vi "GetProbePlanCoordinates.vi"(1 "Probe Card Channels":i32=32) -> (0 "file path":string, 2 "OK?":bool, 3 "Array":T1(array[cluster]))   [LabVIEW 2018]
doc: "Utility to read probe plan from text file and generate respective coordinates in global variable."
uses:
  general_VIs/globals/QC_MeasurementSetup.vi
  ProbePlanParams.vi
  <vilib>/regexp/Match Regular Expression.xnode
panel:
  out "No. probe points":string
  in  "ProbePoints":T2
  out "String":string
  in  "Stop Button":bool
  in  "OK Button":bool
  in  "Region":u16(ring)
  out "Coordinates":string[][](table)
  # "ProbePlan Coordinates"
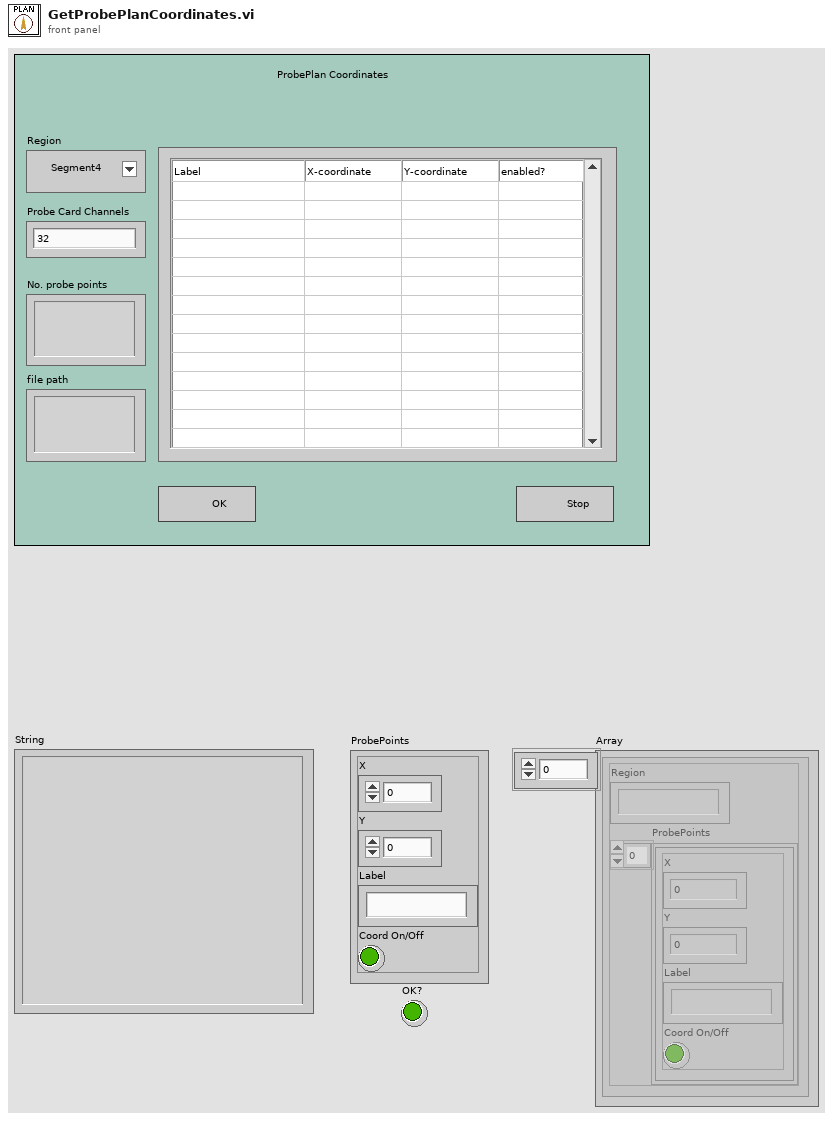
[diagram p1: front panel]
types:
  T1 = cluster{"Region":string, "ProbePoints":cluster{"X":dbl, "Y":dbl, "Label":string, "Coord On/Off":bool}[]}[]
  T2 = cluster{"X":dbl, "Y":dbl, "Label":string, "Coord On/Off":bool}
  T3 = cluster{"Region":string, "ProbePoints":cluster{"X":dbl, "Y":dbl, "Label":string, bool}[]}[]
  T4 = enum16{"open", "replace", "create", "open or create", "replace or create", "replace or create with confirmation"}
  T5 = cluster{"X":dbl, "Y":dbl, "Label":string, bool}[]
  T6 = cluster{"Bias Supply":refnum<class "SupplyControl.lvclass">, "SMU":refnum<class "SupplyControl.lvclass">, "LCR":refnum<class "LCRControl.lvclass">, "ProbeStation":refnum<class "ProbeStationControl.lvclass">, "Arduino":refnum<class "ArduinoControl.lvclass">, "Measurement switch":refnum<class "Switching.lvclass">, "Probe Card Channels":i32, "Bias Voltage [V]":dbl, "First strip":i32, "Last strip":i32, "Base Voltage [V]":dbl, "Base Ramp Step [V]":dbl, "Base Ramp Interval [ms]":u32, "High Voltage [V]":dbl, "High Ramp Step [V]":dbl, "High Ramp Interval [ms]":u32, "AC frequency [Hz]":i32, "AC amplitude [V]":dbl, "RC Configuration":u16, "Single Needle":bool, "Temperature Readout":enum16{"Read Arduino", "Enter manually"}, "Fraction of good strips [%]":dbl, "Measurement switch used?":bool, "Matrix X Channels":cluster{"Mux1 C1":i32, "Mux1 C2":i32, "Mux2 C1":i32, "Mux2 C2":i32}, "Pinholes Y/N":bool, "Capacitance Y/N":bool, "Resistance Y/N":bool, "Bias Supply Name":string, "SMU Name":string, "LCR Name":string}
  T7 = cluster{"result string":string, "ProbePoints":cluster{"X":dbl, "Y":dbl, "Label":string, bool}[]}
  T8 = cluster{"result string":string, "ProbePoints":cluster{"X":dbl, "Y":dbl, "Label":string, bool}[]}[]
  T9 = cluster{"Region":string, "ProbePoints":cluster{"X":dbl, "Y":dbl, "Label":string, bool}[]}
  T10 = cluster{"X":dbl, "Y":dbl, "Label":string, "Coord On/Off":bool}[]
  T11 = cluster{"Region":string, cluster{"X":dbl, "Y":dbl, "Label":string, "Coord On/Off":bool}[]}
  T12 = cluster{"Strip Number OUT":i32, "X0":i32, "Y0":i32, "X1":i32, "Y1":i32, "Xref":dbl, "Yref":dbl, "ProbePlan type":u32, "Inner pads offset":ext, "Outer pads offset":ext, "l_inner":ext, "l_outer":ext, "strip numbering":u16, "Device Orientation":ext, "Stagger offset":i32, "Yoffset":dbl, "Strip pitch":dbl, "Fiducail separation":dbl, "Radius":ext, "Relative strip angles":dbl, "Probeplan description":string, "ProbePlan array":cluster{"Region":string, "ProbePoints":cluster{"X":dbl, "Y":dbl, "Label":string, "CardViable?":bool}[]}[], "Test ProbePoints":cluster{"Regions Enabled":bool[], "From index":u32[], "To index":u32[], "Strip length [cm]":dbl[]}}
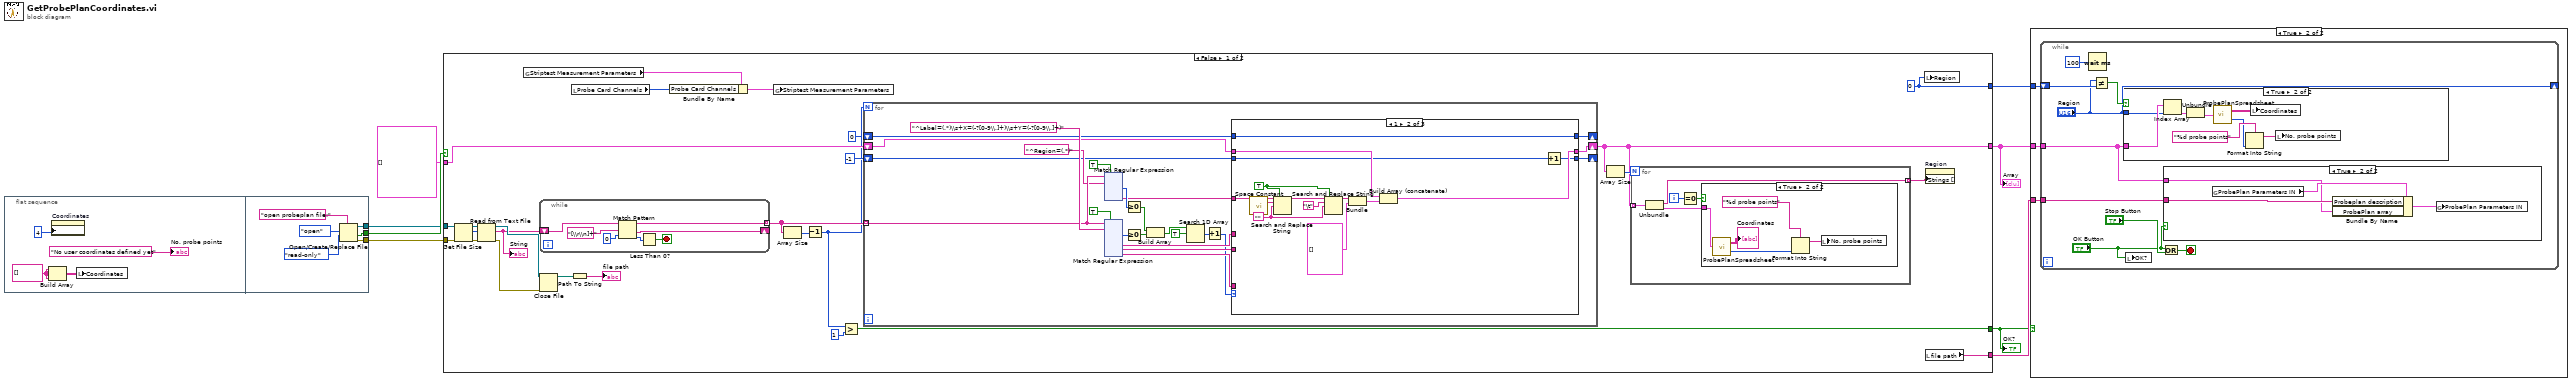
[diagram p0: block diagram]
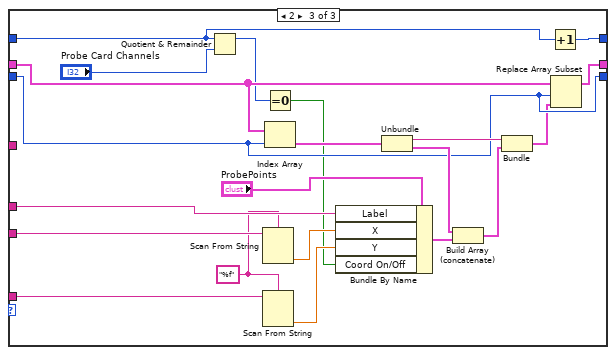
[diagram p7: hidden frame]
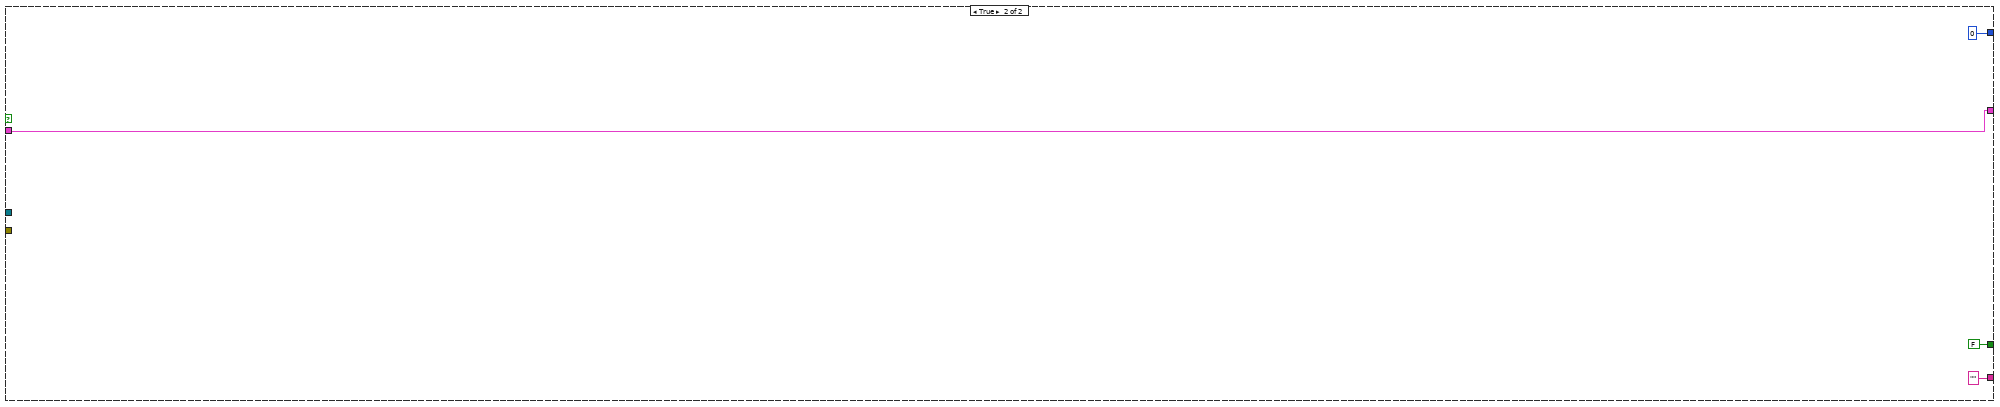
[diagram p8: hidden frame]
diagram:
  n1 = flat-sequence {
    tunnel: [w15] -> w8
    tunnel: [w14] -> w6
    tunnel: [w13] -> w7
    frame #0 {
      w12 = string[] []
      n2 = Build Array(w12, w12, w12) -> (w11:string[][])
      n3 = property on="Coordinates" class="Tbl (strict)"("Number of Columns"=4) -> ()  [unwired: 2 in, 2 out]
      n4 = local write "Coordinates"(w11) -> ()
      "No. probe points" <- "No user coordinates defined yet" ("String 2")
    }
    frame #1 {
      n5 = Open/Create/Replace File(prompt="open probeplan file:", operation (0:open)=T4."open", access (0:read/write)=enum16{"read/write", "read-only", "write-only"}."read-only") -> (refnum out=w13:refnum<file>, cancelled=w15:bool, error out=w14:errorcluster)  [unwired: 3 in]
    }
  }
  n6 = case shown="False" w8 {
    tunnel: T3 [] ("Array") -> [w31 w360]
    tunnel: w7 -> [w44 _]
    tunnel: w6 -> [w39 _]
    tunnel: [w29 w360] -> w4
    tunnel: [w28 0] -> w3
    tunnel: [w24 FALSE] -> w2
    tunnel: [w23 ""] -> w5
    frame False {
      w28 = 0
      n7 = Get File Size(file=w44, error in=w39) -> (refnum out=w43:refnum<file>, size (in bytes)=w38:i64, 0:w41:errorcluster)
      n8 = Read from Text File(file (use dialog)=w43, count=w38, error in=w41) -> (refnum out=w42:refnum<file>, text=w35:string, error out=w40:errorcluster)  [unwired: 1 in, 1 out]
      "String" <- w35
      n9 = global read "QC_MeasurementSetup.vi" "Striptest Measurement Parameters"() -> (w20:T6)
      n10 = while {
        shift-right: [w353] -> _
        shift-left: w35 -> [w356]
        tunnel: [w350] -> w33 mode=indexing
        stop <- w352 stop-if-true
        n11 = Match Pattern(string=w356, regular expression="[\\r\\n]+", offset (0)=0) -> (before substring=w350:string, after substring=w353:string, offset past match=w351:i32)  [unwired: 1 out]
        n12 = Less Than 0?(x=w351) -> (x < 0?=w352:bool)
      }
      n13 = Close File(refnum=w42, error in=w40) -> (path=w37:path)  [unwired: 1 out]
      n14 = Path To String(path=w37) -> (string=→"file path":string)
      n15 = local read "Probe Card Channels"() -> (w21:i32)
      n16 = Bundle By Name(cluster=w20, "Probe Card Channels"=w21) -> (w19:T6)
      n17 = global write "QC_MeasurementSetup.vi" "Striptest Measurement Parameters"(w19) -> ()
      n18 = Array Size(array=w33) -> (size(s)=w34:i32)
      n19 = Decrement(x=w34) -> (x-1=w25:i32)
      n20 = Greater?(x=w25, y=1) -> (0:w24:bool)
      n21 = for {
        N: w25 -> [_]
        tunnel: w33 -> [w71] mode=indexing
        shift-right: [w57] -> _
        shift-left: -1 -> [w58]
        shift-right: [w59] -> w29
        shift-left: w31 -> [w60]
        shift-right: [w56] -> _
        shift-left: 0 -> [w55]
        n22 = xnode "Match Regular Expression"("input string"=w71, "regular expression"="^Region=(.*)", "ignore case? (F)"=TRUE) -> ("offset past match"=w68:i32, "submatch 1"=w61:string)  [unwired: 3 in, 4 out]
        n23 = xnode "Match Regular Expression"("input string"=w71, "regular expression"="^Label=(.*)\\s+X=(-?[0-9\\.]+)\\s+Y=(-?[0-9\\.]+)", "ignore case? (F)"=TRUE) -> ("offset past match"=w74:i32, "submatch 1"=w75:string, "submatch 2"=w72:string, "submatch 3"=w73:string)  [unwired: 3 in, 4 out]
        n24 = Greater Or Equal To 0?(x=w68) -> (x >= 0?=w67:bool)
        n25 = Greater Or Equal To 0?(x=w74) -> (x >= 0?=w66:bool)
        n26 = Build Array(w67, w66) -> (w65:bool[])
        n27 = Search 1D Array(1D array=w65, element=TRUE) -> (index of element=w63:i32)  [unwired: 1 in]
        n28 = Increment(x=w63) -> (x+1=w62:i32)
        n29 = case shown="1" w62 {
          tunnel: w75 -> [_ _ w228]
          tunnel: w73 -> [_ _ w225]
          tunnel: w72 -> [_ _ w227]
          tunnel: w61 -> [_ w203 _]
          tunnel: w60 -> [w196 w209 w220]
          tunnel: [w196 w207 w218] -> w59
          tunnel: w58 -> [w195 w206 w221]
          tunnel: [w195 w205 w221] -> w57
          tunnel: [w194 w204 w212] -> w56
          tunnel: w55 -> [w194 w204 w211]
          frame 0, Default {
          }
          frame 1 {
            w197 = TRUE
            w198 = ""
            n30 = call <vilib>:"Space Constant.vi"() -> ("String"=w202:string)
            n31 = Search and Replace String(replace all?=w197, input string=w203, search string=w202, replace string=w198) -> (result string=w201:string)  [unwired: 4 in, 3 out]
            n32 = Search and Replace String(replace all?=w197, input string=w201, search string="\t", replace string=w198) -> (result string=w200:string)  [unwired: 4 in, 3 out]
            n33 = Bundle("result string"=w200, "ProbePoints"=T5 []) -> (w208:T7)  [unwired: 1 in]
            n34 = Build Array (concatenate)(w209, w208) -> (w207:T8)
            n35 = Increment(x=w206) -> (x+1=w205:i32)
          }
          frame 2 {
            w224 = "%f" ("format string")
            n36 = Quotient & Remainder(x=w211, y="Probe Card Channels") -> (x-y*floor(x/y)=w215:i32)  [unwired: 1 out]
            n37 = Scan From String(format string=w224, input string=w227) -> (output 1=w226:dbl)  [unwired: 3 in, 3 out]
            n38 = Scan From String(format string=w224, input string=w225) -> (output 1=w223:dbl)  [unwired: 3 in, 3 out]
            n39 = Equal To 0?(x=w215) -> (x = 0?=w213:bool)
            n40 = Index Array(array=w220, index=w221) -> (element=w231:T9)
            n41 = Bundle By Name(cluster="ProbePoints", "Label"=w228, "X"=w226, "Y"=w223, "Coord On/Off"=w213) -> (w216:T2)
            n42 = Unbundle(w231) -> ("Region"=w230:string, "ProbePoints"=w229:T5)
            n43 = Build Array (concatenate)(w229, w216) -> (w222:T10)
            n44 = Bundle("Region"=w230, w222) -> (w219:T11)  [unwired: 1 in]
            n45 = Increment(x=w211) -> (x+1=w212:i32)
            n46 = Replace Array Subset(array=w220, new element=w219, index=w221) -> (w218:T3)
          }
        }
      }
      n47 = Array Size(array=w29) -> (size(s)=w30:i32)
      n48 = for {
        N: w30 -> [_]
        tunnel: w29 -> [w49] mode=indexing
        tunnel: [w48] -> w27 mode=indexing
        i -> [w46]
        n49 = Unbundle(w49) -> ("Region"=w48:string, "ProbePoints"=w47:T5)
        n50 = Equal To 0?(x=w46) -> (x = 0?=w45:bool)
        n51 = case shown="True" w45 {
          tunnel: w47 -> [_ w52]
          frame False {
          }
          frame True {
            n52 = call "ProbePlanSpreadsheet.vi"("ProbePoints"=w52) -> ("Coordinates"=→"Coordinates":string[][], "Number of ProbePoints"=w51:i32)
            n53 = Format Into String(format string="%d probe points", w51) -> (resulting string=w53:string)  [unwired: 2 in, 1 out]
            n54 = local write "No. probe points"(w53) -> ()
          }
        }
      }
      n55 = local write "Region"(w28) -> ()
      n56 = property on="Region" class="Ring (strict)"("Strings []"=w27) -> ()  [unwired: 2 in, 2 out]
      n57 = local read "file path"() -> (w23:string)
    }
    frame True {
    }
  }
  "Array" <- w4
  "OK?" <- w2
  n58 = case shown="True" w2 {
    tunnel: w3 -> [_ w363]
    tunnel: w4 -> [_ w362]
    tunnel: w5 -> [_ w361]
    frame False {
    }
    frame True {
      n59 = while {
        shift-right: ["Region"] -> _
        shift-left: w363 -> [w371]
        tunnel: w362 -> [w368]
        tunnel: w361 -> [w367]
        stop <- w372 stop-if-true
        n60 = Wait (ms)(milliseconds to wait=u32 100) -> ()  [unwired: 1 out]
        n61 = Not Equal?(x="Region", y=w371) -> (x != y?=w370:bool)
        n62 = case shown="True" w370 {
          tunnel: w368 -> [_ w384]
          tunnel: "Region" -> [_ w382]
          frame False {
          }
          frame True {
            n63 = Index Array(array=w384, index=w382) -> (element=w383:T9)
            n64 = Unbundle(w383) -> ("ProbePoints"=w379:T5)  [unwired: 1 out]
            n65 = call "ProbePlanSpreadsheet.vi"("ProbePoints"=w379) -> ("Coordinates"=w377:string[][], "Number of ProbePoints"=w378:i32)
            n66 = Format Into String(format string="%d probe points", w378) -> (resulting string=w381:string)  [unwired: 2 in, 1 out]
            n67 = local write "Coordinates"(w377) -> ()
            n68 = local write "No. probe points"(w381) -> ()
          }
        }
        n69 = local write "OK?"("OK Button") -> ()
        n70 = Or(x="OK Button", y="Stop Button") -> (x .or. y?=w372:bool)
        n71 = case shown="True" "OK Button" {
          tunnel: w368 -> [_ w373]
          tunnel: w367 -> [_ w374]
          frame False {
          }
          frame True {
            n72 = global read "ProbePlanParams.vi" "ProbePlan Parameters IN"() -> (w376:T12)
            n73 = Bundle By Name(cluster=w376, "Probeplan description"=w374, "ProbePlan array"=w373) -> (w375:T12)
            n74 = global write "ProbePlanParams.vi" "ProbePlan Parameters IN"(w375) -> ()
          }
        }
      }
    }
  }
